vi "GeneratePlaneEquation.vi"(8 "Error In":errorcluster, 11 "Three  points":dbl[][](array[numeric])) -> (0 "Error Out":errorcluster, 1 "Equation":string, 2 "D":dbl, 3 "NormalVector":dbl[](array[numeric]))   [LabVIEW 2019]
uses:
  <vilib>/Analysis/baseanly.llb/Real Dot Product.vi
  <vilib>/Analysis/NI_AALBase.lvlib
  <vilib>/Analysis/NI_AALPro.lvlib
panel:
  out "Counter2":i32
  out "Counter":i32
  out "V2":dbl[](array[numeric])
  out "V1":dbl[](array[numeric])
  # "This Vi generates a plane equation from 3 given initial points"
  # "Ax + By + Cz = <A,B,C> . <X_0,Y_0,Z_0> = D"
  # "Nx"
  # "Ny"
  # "Nz"
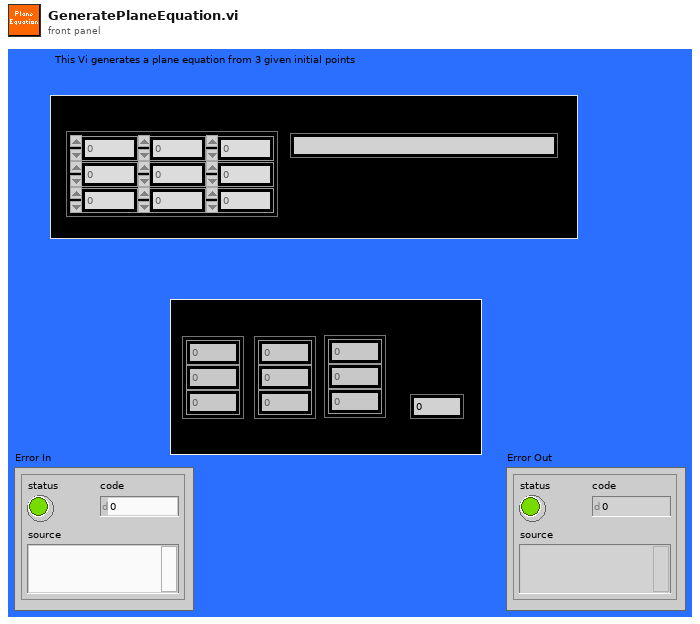
[diagram p1: front panel]
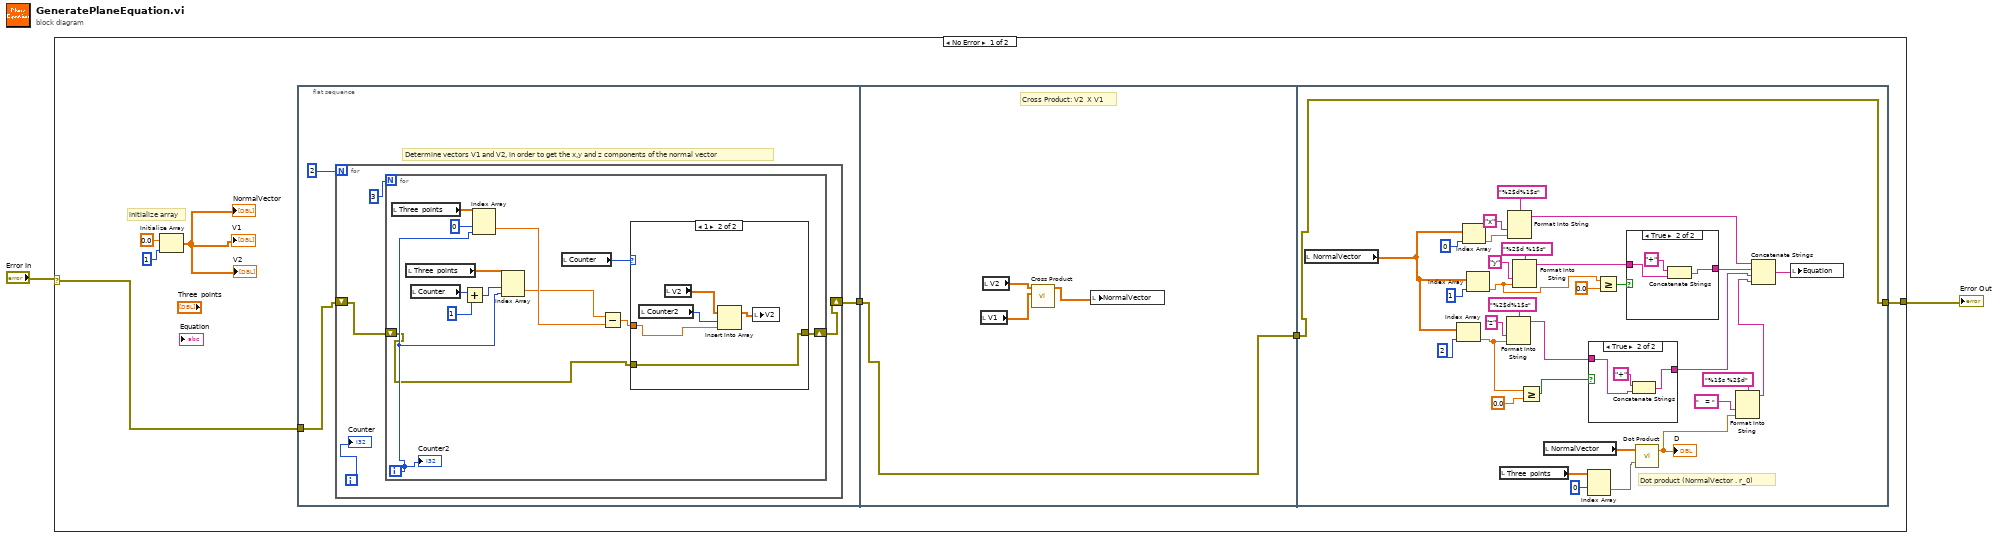
[diagram p0: block diagram]
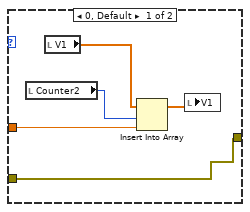
[diagram p2: hidden frame]
diagram:
  n1 = case shown="No Error" "Error In" {
    selector: "Error In" -> [w6 w84]
    tunnel: [w3 w84] -> w1
    frame No Error {
      # "initialize array"
      n2 = Initialize Array(0.0 ("element"), 1 ("dimension size")) -> (→"NormalVector" →"V1" →"V2":dbl[])
      n3 = flat-sequence {
        tunnel: w6 -> [w11]
        tunnel: [w10] -> w5
        tunnel: w5 -> [w43]
        tunnel: [w43] -> w4
        tunnel: w4 -> [w44]
        tunnel: [w44] -> w3
        frame #0 {
          # "Determine vectors V1 and V2, in order to get the x,y and z components of the normal vector"
          n4 = for {
            N: 2 -> [_]
            shift-right: [w13] -> w10
            shift-left: w11 -> [w14]
            i -> [w15]
            n5 = for {
              N: 3 -> [_]
              shift-right: [w17] -> w13
              shift-left: w14 -> [w18]
              i -> [w21]
              n6 = local read "Three  points"() -> (w29:dbl[][])
              n7 = local read "Three  points"() -> (w26:dbl[][])
              n8 = local read "Counter"() -> (w25:i32)
              n9 = Add(x=w25, y=1) -> (x+y=w23:i32)
              n10 = Index Array(array=w29, index (row)=0, index (col)=w21) -> (element=w22:dbl)
              n11 = Index Array(array=w26, index (row)=w23, index (col)=w21) -> (element=w19:dbl)
              n12 = local read "Counter"() -> (w27:i32)
              n13 = Subtract(x=w19, y=w22) -> (x-y=w20:dbl)
              n14 = case shown="1" w27 {
                tunnel: w20 -> [w32 w36]
                tunnel: w18 -> [w30 w35]
                tunnel: [w30 w35] -> w17
                frame 0, Default {
                  n15 = local read "Counter2"() -> (w31:i32)
                  n16 = local read "V1"() -> (w33:dbl[])
                  n17 = Insert Into Array(array=w33, index=w31, new element=w32) -> (w34:dbl[])
                  n18 = local write "V1"(w34) -> ()
                }
                frame 1 {
                  n19 = local read "Counter2"() -> (w37:i32)
                  n20 = local read "V2"() -> (w38:dbl[])
                  n21 = Insert Into Array(array=w38, index=w37, new element=w36) -> (w39:dbl[])
                  n22 = local write "V2"(w39) -> ()
                }
              }
              "Counter2" <- w21
            }
            "Counter" <- w15
          }
        }
        frame #1 {
          # "Cross Product: V2  X V1"
          n23 = local read "V1"() -> (w42:dbl[])
          n24 = local read "V2"() -> (w41:dbl[])
          n25 = call <vilib>:"Cross Product.vi"("B Vector"=w42, "A Vector"=w41) -> ("Cross Product"=w40:dbl[])  [unwired: 8 in, 1 out]
          n26 = local write "NormalVector"(w40) -> ()
        }
        frame #2 {
          # "Dot product (NormalVector . r_0)"
          n27 = local read "NormalVector"() -> (w68:dbl[])
          n28 = Index Array(array=w68, index=2) -> (element=w52:dbl)
          n29 = Index Array(array=w68, index=0) -> (element=w49:dbl)
          n30 = Index Array(array=w68, index=1) -> (element=w53:dbl)
          n31 = local read "Three  points"() -> (w74:dbl[][])
          n32 = Format Into String(format string="%2$d%1$s", "z" ("initial string"), w52) -> (resulting string=w62:string)  [unwired: 2 in, 1 out]
          n33 = Format Into String(format string="%2$d%1$s", "x" ("initial string"), w49) -> (resulting string=w61:string)  [unwired: 2 in, 1 out]
          n34 = Format Into String(format string="%2$d %1$s", "y" ("initial string"), w53) -> (resulting string=w63:string)  [unwired: 2 in, 1 out]
          n35 = Greater Or Equal?(x=w52, y=0.0) -> (x >= y?=w65:bool)
          n36 = local read "NormalVector"() -> (w75:dbl[])
          n37 = Index Array(array=w74, index (row)=0) -> (element=w72:dbl[])  [unwired: 1 in]
          n38 = case shown="True" w65 {
            tunnel: w62 -> [w76 w78]
            tunnel: [w76 w77] -> w59
            frame False {
            }
            frame True {
              n39 = Concatenate Strings("+" ("string"), w78) -> (w77:string)
            }
          }
          n40 = Greater Or Equal?(x=w53, y=0.0) -> (x >= y?=w66:bool)
          n41 = case shown="True" w66 {
            tunnel: w63 -> [w80 w82]
            tunnel: [w80 w81] -> w60
            frame False {
            }
            frame True {
              n42 = Concatenate Strings("+" ("string"), w82) -> (w81:string)
            }
          }
          n43 = call-poly <vilib>:"Dot Product.vi"("Y Vector"=w72, "X Vector"=w75) -> ("X * Y"=w45:dbl)  [unwired: 1 out]
          "D" <- w45
          n44 = Format Into String(format string="%1$s %2$d", "   = " ("initial string"), w45) -> (resulting string=w58:string)  [unwired: 2 in, 1 out]
          n45 = Concatenate Strings(w61, w60, w59, w58) -> (w57:string)
          n46 = local write "Equation"(w57) -> ()
        }
      }
    }
    frame Error {
    }
  }
  "Error Out" <- w1
